vi "pid控制-静止.vi"(0 "目标p1":dbl, 1 "当前p1":dbl, 2 "kp1":dbl, 3 "ki1":dbl, 4 "kd1":dbl, 5 "目标p2":dbl, 6 "当前p2":dbl, 7 "kp2":dbl, 8 "ki2":dbl, 9 "kd2":dbl) -> (10 "输出v":dbl)   [LabVIEW 2022 SP3]
panel:
  out "OUT2":dbl
  out "OUT1":dbl
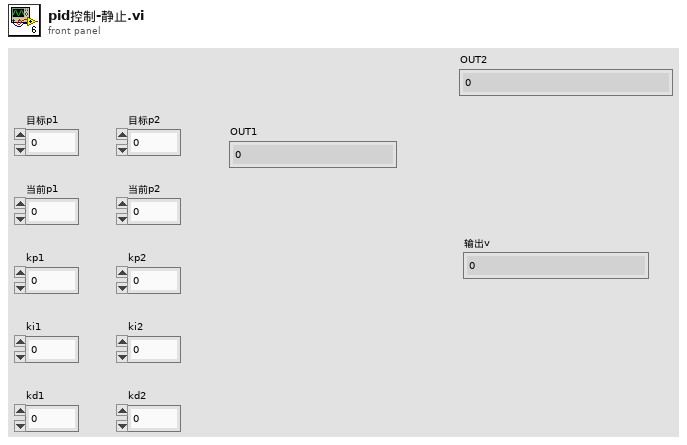
[diagram p1: front panel]
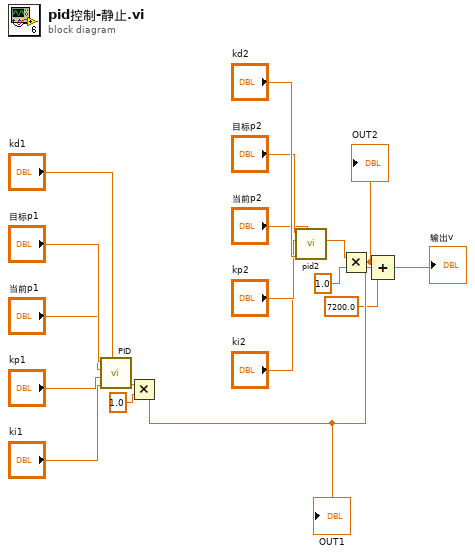
[diagram p0: block diagram]
diagram:
  n1 = call "PID.vi"("目标"="目标p1", "当前"="当前p1", "kp"="kp1", "ki"="ki1", "kd"="kd1") -> ("out"=w18:dbl)
  n2 = Multiply(x=w18, y=1.0) -> (x*y=w14:dbl)
  "OUT1" <- w14
  n3 = call "pid2.vi"("当前"="当前p2", "kd"="kd2", "ki"="ki2", "kp"="kp2", "目标"="目标p2") -> ("out"=w1:dbl)  [unwired: 6 in]
  n4 = Multiply(x=w1, y=1.0) -> (x*y=w15:dbl)
  "OUT2" <- w15
  n5 = Compound Arithmetic op=ADD(w15, w14, 7200.0 ("值")) -> (→"输出v":dbl)
